vi "Log The Message.vi"(11 "Reset Message":refnum<class "Reset Message.lvclass">) -> (2 "log text":string="Reset Image")   [LabVIEW 2023, in "Draw Messages.lvlib" / "Reset Message.lvclass"]
uses:
  Reset Message.lvclass
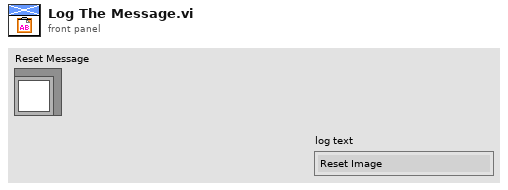
[diagram p1: front panel]
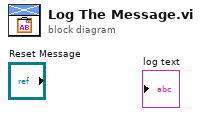
[diagram p0: block diagram]
diagram:
